vi "Create Message Data Clusters.vi"(7 "Message parameters":T1[](array[typedef]), 8 "error in (no error)":errorcluster, 11 "Server class in":refnum<vi>) -> (0 "error out":errorcluster, 3 "Server class out":refnum<vi>)   [LabVIEW 2019, in "gRPC Scripting Tools.lvlib"]
uses:
  gRPC Scripting Tools.lvlib
  TypeDefs/Message Metadata (Scripting).ctl
  TypeDefs/Message Element Metadata (Scripting).ctl
  TypeDefs/Message Element Type.ctl
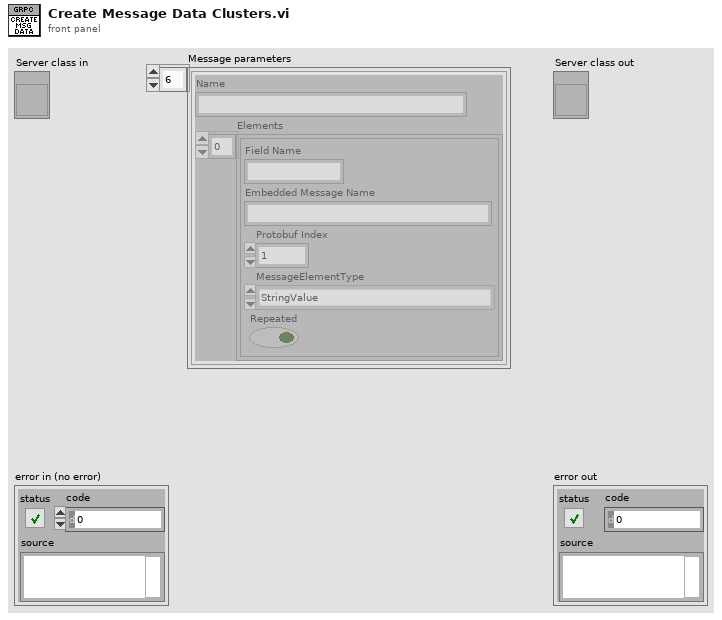
[diagram p1: front panel]
types:
  T1 = typedef "gRPC Scripting Tools.lvlib/Message Metadata (Scripting).ctl" = cluster{"Name":string, "Elements":T2[]}
  T2 = typedef "gRPC Scripting Tools.lvlib/Message Element Metadata (Scripting).ctl" = cluster{"Field Name":string, "Embedded Message Name":string, "Protobuf Index":i32, "MessageElementType":T3, "Repeated":bool}
  T3 = typedef "gRPC Scripting Tools.lvlib/Message Element Type.ctl" = enum32{"Int32Value", "FloatValue", "DoubleValue", "BoolValue", "StringValue", "MessageValue", ""}
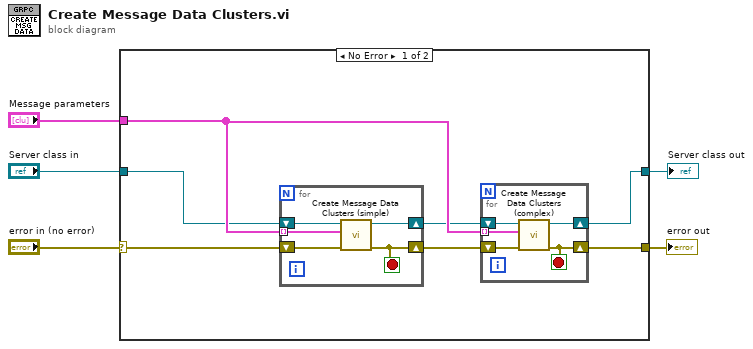
[diagram p0: block diagram]
diagram:
  n1 = case shown="No Error" "error in (no error)" {
    selector: "error in (no error)" -> [w6 w23]
    tunnel: "Message parameters" -> [w12 _]
    tunnel: [w11 w24] -> w4
    tunnel: [w9 w23] -> w3
    tunnel: "Server class in" -> [w7 w24]
    frame No Error {
      n2 = for {
        shift-right: [w20] -> w8
        shift-left: w7 -> [w22]
        shift-right: [w18] -> w10
        shift-left: w6 -> [w21]
        tunnel: w12 -> [w19] mode=indexing
        stop <- w18 stop-if-true
        n3 = call "Create Message Data Clusters (simple).vi"("error in (no error)"=w21, "Message Metadata"=w19, "LVClassLibrary in"=w22) -> ("error out"=w18:errorcluster, "LVClassLibrary out"=w20:refnum<vi>)  [unwired: 7 in]
      }
      n4 = for {
        shift-right: [w15] -> w11
        shift-left: w8 -> [w17]
        shift-right: [w13] -> w9
        shift-left: w10 -> [w16]
        tunnel: w12 -> [w14] mode=indexing
        stop <- w13 stop-if-true
        n5 = call "Create Message Data Clusters (complex).vi"("error in (no error)"=w16, "Message Metadata"=w14, "LVClassLibrary in"=w17) -> ("error out"=w13:errorcluster, "LVClassLibrary out"=w15:refnum<vi>)  [unwired: 7 in]
      }
    }
    frame Error {
    }
  }
  "Server class out" <- w4
  "error out" <- w3
